vi "Event Log.Record Event.vi"(8 "error in":errorcluster, 10 "Message":string) -> (0 "error out":errorcluster)   [LabVIEW 2024, in "EQMF.lvlib" / "Event Log.lvlib"]
uses:
  Event Log.lvlib
  Queues/Queue Utils.lvlib
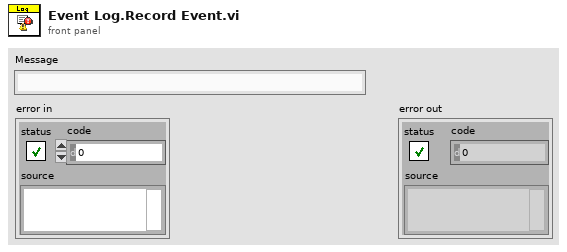
[diagram p1: front panel]
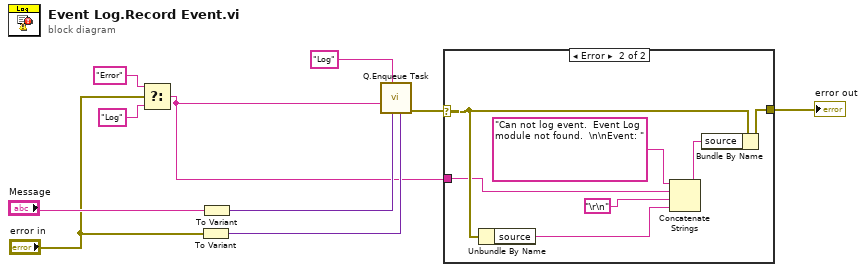
[diagram p0: block diagram]
diagram:
  n1 = Select(t="Error" ("Cmd"), s="error in", f="Log" ("Cmd")) -> (s? t:f=w1:string)
  n2 = To Variant(anything="error in") -> (Variant=w5:variant)
  n3 = To Variant(anything="Message") -> (Variant=w4:variant)
  n4 = call "Q.Enqueue Task.vi"("Data2"=w5, "Data1"=w4, "Q Name"="Log" ("name (unnamed)"), "Task Name"=w1) -> ("error out"=w2:errorcluster)  [unwired: 6 in, 1 out]
  n5 = case shown="Error" w2 {
    selector: w2 -> [w11 w17]
    tunnel: [w11 w18] -> w3
    tunnel: w1 -> [_ w14]
    frame No Error {
    }
    frame Error {
      n6 = Unbundle By Name(w17) -> ("source"=w12:string)
      n7 = Concatenate Strings("Can not log event.  Event Log module not found.  \n\nEvent: ", w14, "\r\n", w12) -> (w16:string)
      n8 = Bundle By Name(cluster=w17, "source"=w16) -> (w18:errorcluster)
    }
  }
  "error out" <- w3
